vi "Rename Object Labels.vi"(6 "Post":string, 7 "Traverse Target":T1, 8 "error in":errorcluster, 9 "Pre":string, 10 "Class Ref":refnum<vi>) -> (0 "error out":errorcluster)   [LabVIEW 2021, in "_Rename.lvlib" / "_Rename.lvclass"]
uses:
  _Rename.lvclass
  _Rename.lvclass/_Rename.ctl
  <vilib>/Utility/traverseref.llb/TRef TravTarget.ctl
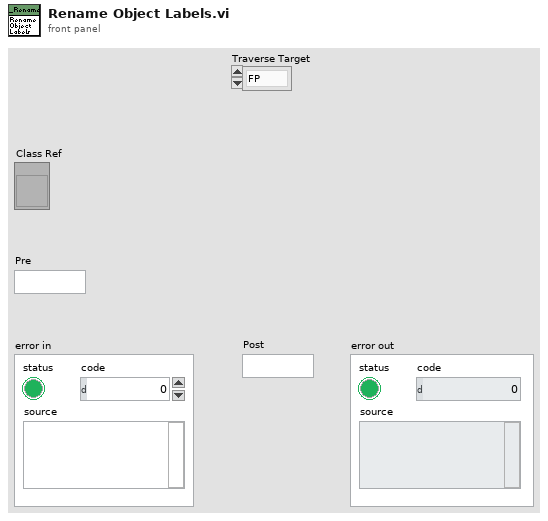
[diagram p1: front panel]
types:
  T1 = typedef "TRef TravTarget.ctl" = enum16{"FP", "BD", "Other"}
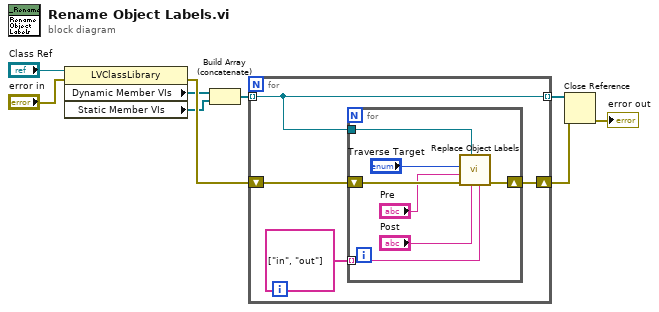
[diagram p0: block diagram]
diagram:
  n1 = property class="LVClassLibrary"(reference="Class Ref", error in="error in") -> (error out=w9:errorcluster, "Dynamic Member VIs"=w6:refnum<vi>[], "Static Member VIs"=w7:refnum<vi>[])  [unwired: 1 out]
  n2 = Build Array (concatenate)(w6, w7) -> (w8:refnum<vi>[])
  n3 = for {
    tunnel: w8 -> [w11] mode=indexing
    shift-right: [w10] -> w4
    shift-left: w9 -> [w13]
    tunnel: [w11] -> w5 mode=indexing
    n4 = for {
      tunnel: w11 -> [w19]
      tunnel: string[] ["in", "out"] -> [w17] mode=indexing
      shift-right: [w16] -> w10
      shift-left: w13 -> [w18]
      n5 = call "Replace Object Labels.vi"("in / out"=w17, "Post"="Post", "VI Ref"=w19, "error in"=w18, "Pre"="Pre", "Traverse Target"="Traverse Target") -> ("error out"=w16:errorcluster)  [unwired: 5 in]
    }
  }
  n6 = Close Reference(reference=w5, error in (no error)=w4) -> (error out=→"error out":errorcluster)
